vi "Combine Images Vertically.vi"(8 "Error In":errorcluster, 11 "Paths to images in":path[](array[path])) -> (0 "Error Out":errorcluster, 3 "Paths to images out":path[](array[path]))   [LabVIEW 2014, in "i3-docs.lvlib"]
uses:
  i3-docs.lvlib
  <vilib>/printing/ReportDocExtensions.llb/File_types_for_reports.ctl
  <vilib>/wsapi/NI_WebServices.lvlib
  <vilib>/Utility/NIReport.llb/NI_ReportGenerationCore.lvlib
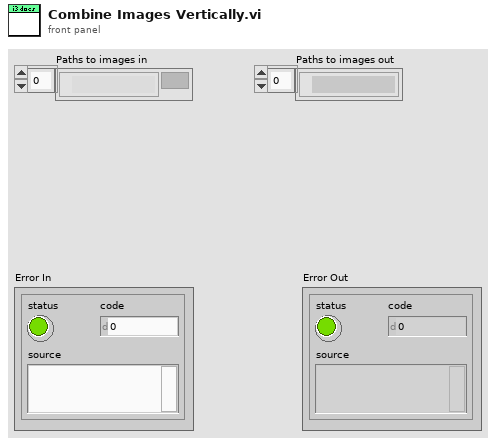
[diagram p1: front panel]
types:
  T1 = typedef "NI_ReportGenerationCore.lvlib/File_types_for_reports.ctl" = enum16{".jpg", ".png", ".html", ".gif"}
  T2 = enum16{"open", "replace", "create", "open or create", "replace or create", "replace or create with confirmation"}
  T3 = typedef "imagedata.ctl" = cluster{"image type":i32, "image depth":i32, "image":u8[], "mask":u8[], "colors":u32[], "Rectangle":cluster{"left":i16, "top":i16, "right":i16, "bottom":i16}}
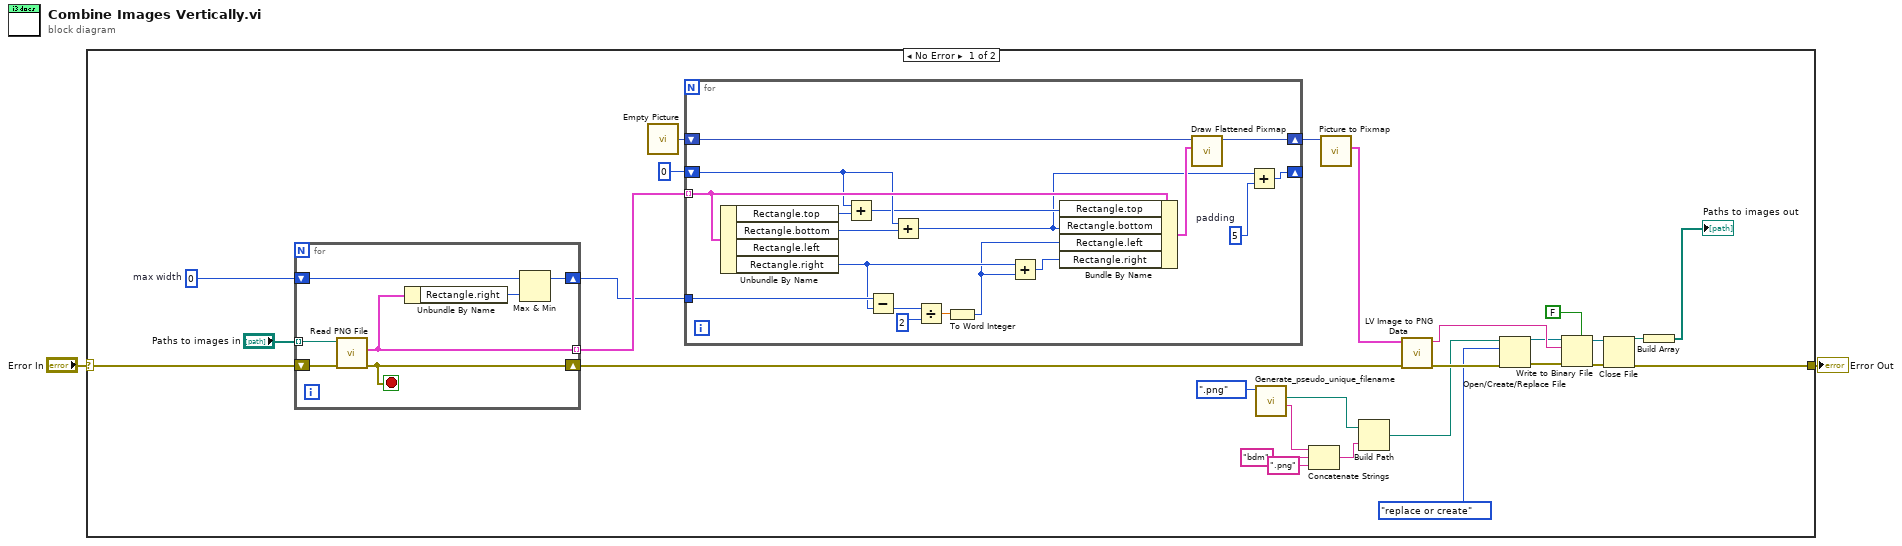
[diagram p0: block diagram]
diagram:
  n1 = case shown="No Error" "Error In" {
    selector: "Error In" -> [w30 w56]
    tunnel: [w13 w56] -> w1
    frame No Error {
      w29 = i16 0  # max width
      n2 = for {
        shift-right: [w54] -> w23
        shift-left: w30 -> [w55]
        shift-right: [w50] -> w25
        shift-left: w29 -> [w52]
        tunnel: [w53] -> w28 mode=indexing
        tunnel: "Paths to images in" -> [w49] mode=indexing
        stop <- w54 stop-if-true
        n3 = call <vilib>:"Read PNG File.vi"("error in (no error)"=w55, "path to PNG file"=w49) -> ("error out"=w54:errorcluster, "image data"=w53:T3)  [unwired: 7 in, 1 out]
        n4 = Unbundle By Name(w53) -> ("Rectangle.right"=w51:i16)
        n5 = Max & Min(x=w52, y=w51) -> (max(x,y)=w50:i16)  [unwired: 1 out]
      }
      n6 = call "Empty Picture"() -> ("empty picture"=w27:picture)
      n7 = for {
        tunnel: w28 -> [w46] mode=indexing
        shift-right: [w48] -> w24
        shift-left: w27 -> [w47]
        shift-right: [w35] -> _
        shift-left: i16 0 -> [w43]
        tunnel: w25 -> [w40]
        w33 = i16 5  # padding
        n8 = Unbundle By Name(w46) -> ("Rectangle.top"=w45:i16, "Rectangle.bottom"=w42:i16, "Rectangle.right"=w37:i16)  [unwired: 1 out]
        n9 = Add(x=w43, y=w45) -> (x+y=w41:i16)
        n10 = Subtract(x=w40, y=w37) -> (x-y=w39:i16)
        n11 = Add(x=w43, y=w42) -> (x+y=w34:i16)
        n12 = Divide(x=w39, y=2) -> (x/y=w32:dbl)
        n13 = To Word Integer(number=w32) -> (16bit integer=w31:i16)
        n14 = Add(x=w37, y=w31) -> (x+y=w36:i16)
        n15 = Bundle By Name(cluster=w46, "Rectangle.top"=w41, "Rectangle.bottom"=w34, "Rectangle.left"=w31, "Rectangle.right"=w36) -> (w44:T3)
        n16 = call <vilib>:"Draw Flattened Pixmap.vi"("image data"=w44, "picture"=w47) -> ("new picture"=w48:picture)  [unwired: 7 in]
        n17 = Add(x=w34, y=w33) -> (x+y=w35:i16)
      }
      n18 = call <vilib>:"Generate_pseudo_unique_filename.vi"("file type(.jpg)"=File_types_for_reports.".png") -> ("root filename"=w6:string, "temp directory"=w8:path)  [unwired: 8 in, 1 out]
      n19 = Concatenate Strings(w6, "bdm" ("string"), ".png" ("string")) -> (w7:string)
      n20 = call <vilib>:"Picture to Pixmap.vi"("picture"=w24) -> ("image data"=w22:T3)  [unwired: 9 in, 1 out]
      n21 = Build Path(base path=w8, name or relative path=w7) -> (appended path=w3:path)
      n22 = call <vilib>:"LV Image to PNG Data.vi"("error in (no error)"=w23, "image data"=w22) -> ("error out"=w20:errorcluster, "png data"=w17:string)  [unwired: 8 in]
      n23 = Open/Create/Replace File(file path (use dialog)=w3, error in=w20, operation (0:open)=T2."replace or create") -> (refnum out=w16:refnum<file>, error out=w15:errorcluster)  [unwired: 3 in, 1 out]
      n24 = Write to Binary File(file (use dialog)=w16, data=w17, error in=w15, 5:FALSE ("prepend array or string size? (T)")) -> (refnum out=w12:refnum<file>, error out=w14:errorcluster)  [unwired: 2 in, 1 out]
      n25 = Close File(refnum=w12, error in=w14) -> (path=w11:path, error out=w13:errorcluster)
      n26 = Build Array(w11) -> (→"Paths to images out":path[])
    }
    frame Error {
    }
  }
  "Error Out" <- w1
